vi "Grab SSID Values.vi"(8 "error in (no error)":errorcluster, 11 "standard output":string="SSID 1 : \n    Network type            : Infrastructure\r\n    Authentication          : WPA2-Personal\r\n    Encryption              : CCMP \r\n\r\nSSID 2 : MONU_SIGN_HUB\r\n    Network type            : Infrastructure\r\n    Authentication          : WPA2-Personal\r\n    Encryption              : CCMP \r\n\r\nSSID 3 : UHS-GUEST\r\n    Network type            : Infrastructure\r\n    Authentication          : WPA2-Personal\r\n    Encryption              : CCMP \r\n\r\nSSID 4 : UHS\r\n    Network type            : Infrastructure\r\n    Authentication          : Open\r\n    Encryption              : CCMP \r\n\r\nSSID 5 : MB Hotspot 66929\r\n    Network type            : Infrastructure\r\n    Authentication          : WPA2-Personal\r\n    Encryption              : CCMP \r\n\r\nSSID 6 : MYCAR6741\r\n    Network type            : Infrastructure\r\n    Authentication          : WPA2-Personal\r\n    Encryption              : CCMP \r\n\r\nSSID 7 : Justinƒ?Ts iPhone\r\n    Network type            : Infrastructure\r\n    Authentication          : WPA2-Personal\r\n    Encryption              : CCMP \r\n\r\nSSID 8 : \r\n    Network type            : Infrastructure\r\n    Authentication          : Open\r\n    Encryption              : None \r\n\r\nSSID 9 : InDemand\r\n    Network type            : Infrastructure\r\n    Authentication          : Open\r\n    Encryption              : CCMP \r\n\r\nSSID 10 : RTC-Transit-VLAN\r\n    Network type            : Infrastructure\r\n    Authentication          : WPA2-Personal\r\n    Encryption              : CCMP \r\n\r\n") -> (0 "error out":errorcluster, 1 "SSID Count":i32=9, 3 "SSID Values":T1[](array[typedef])=[{"SSID"="Network", "Pswd?"=FALSE, "Hide?"=FALSE}, {"SSID"="MONU_SIGN_HUB", "Pswd?"=FALSE, "Hide?"=FALSE}, {"SSID"="UHS-GUEST", "Pswd?"=FALSE, "Hide?"=FALSE}, {"SSID"="UHS", "Pswd?"=FALSE, "Hide?"=FALSE}, {"SSID"="MB", "Pswd?"=FALSE, "Hide?"=FALSE}, {"SSID"="MYCAR6741", "Pswd?"=FALSE, "Hide?"=FALSE}, {"SSID"="Justinƒ?Ts", "Pswd?"=FALSE, "Hide?"=FALSE}, {"SSID"="InDemand", "Pswd?"=TRUE, "Hide?"=FALSE}, {"SSID"="RTC-Transit-VLAN", "Pswd?"=FALSE, "Hide?"=FALSE}])   [LabVIEW 2024]
uses:
  Controls/Network.ctl
  <vilib>/Utility/error.llb/Trim Whitespace One-Sided.vi
panel:
  out "length":i32
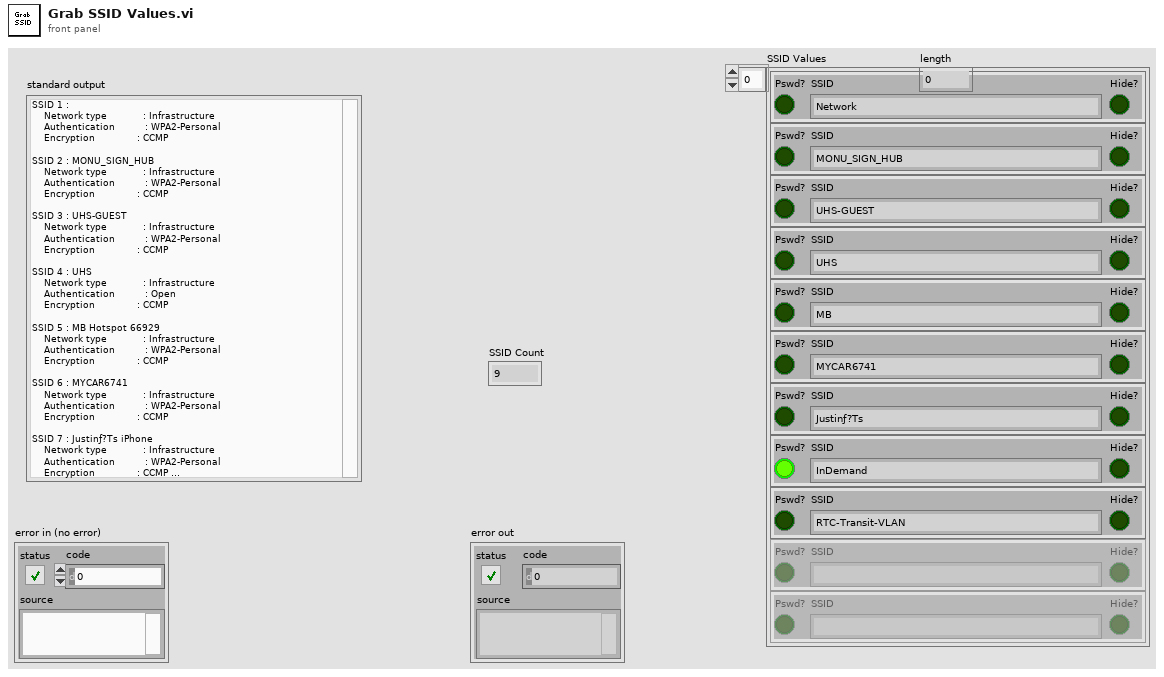
[diagram p1: front panel]
types:
  T1 = typedef "Network.ctl" = cluster{"SSID":string, "Pswd?":bool, "Hide?":bool}
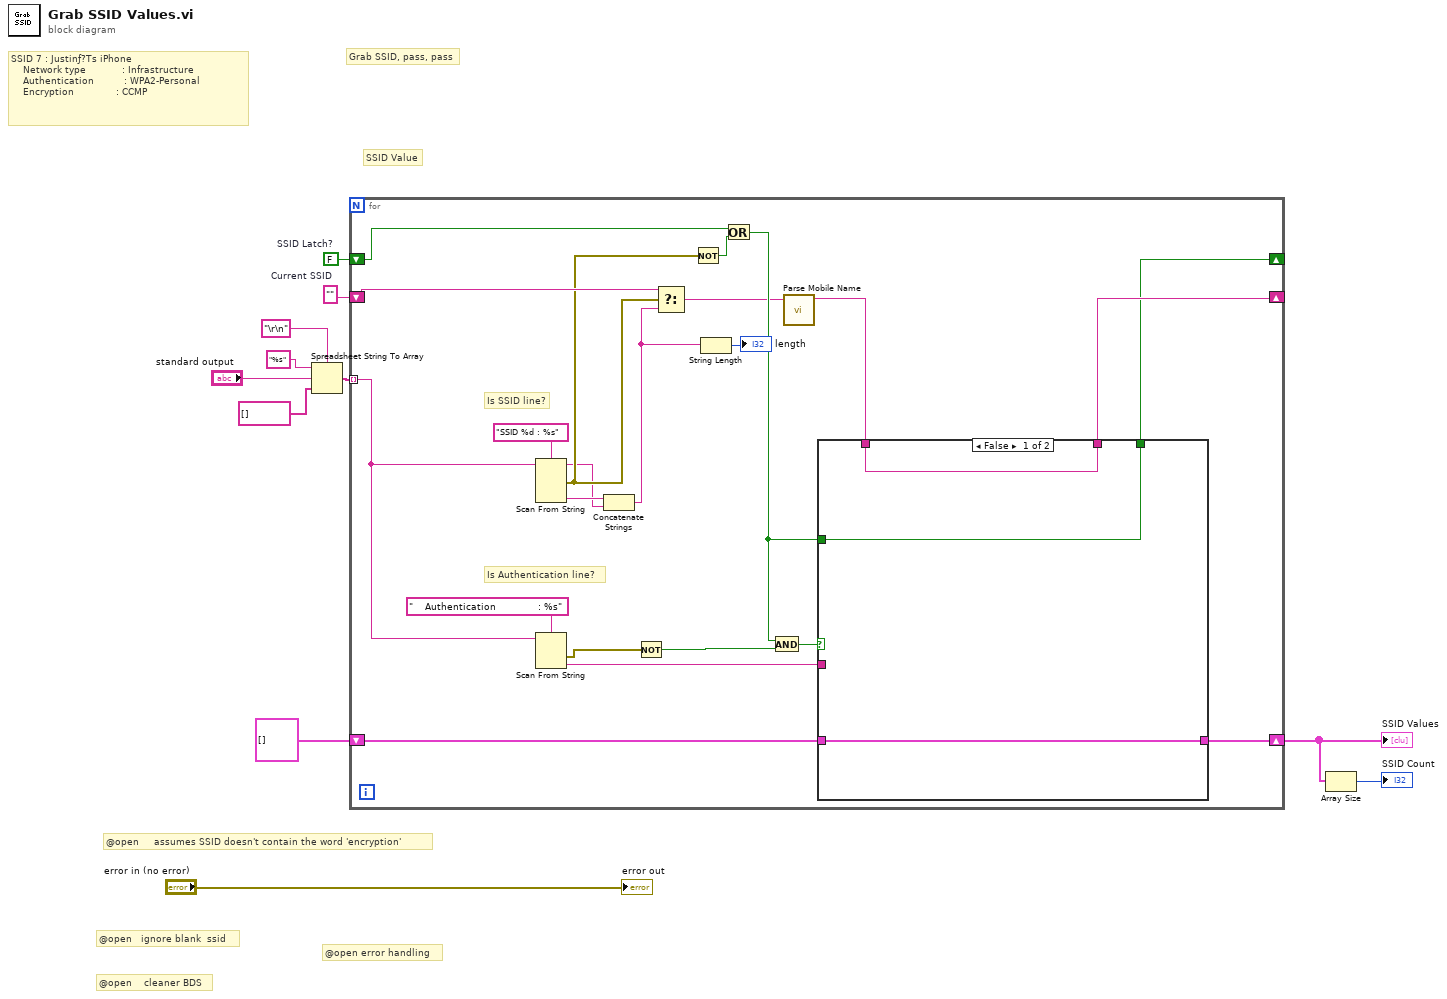
[diagram p0: block diagram]
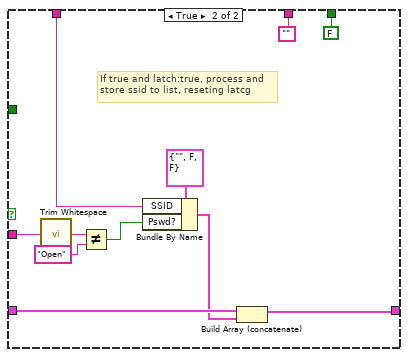
[diagram p2: hidden frame]
diagram:
  w5 = FALSE  # SSID Latch?
  w6 = ""  # Current SSID
  # "@open    cleaner BDS"
  # "@open error handling"
  # "@open   ignore blank  ssid"
  # "@open     assumes SSID doesn't contain the word 'encryption'"
  # "SSID Value"
  # "Grab SSID, pass, pass"
  # "SSID 7 : Justinƒ?Ts iPhone\n    Network type            : Infrastructure\n    Authentication          : WPA2-Personal\n    Encryption              : CCMP"
  n1 = Spreadsheet String To Array(delimiter (Tab)="\r\n", format string="%s", spreadsheet string="standard output", array type (2D Dbl)=string[] []) -> (array=w4:string[])
  n2 = for {
    shift-right: [w27] -> _
    shift-left: w6 -> [w23]
    shift-right: [w26] -> _
    shift-left: w5 -> [w24]
    tunnel: w4 -> [w31] mode=indexing
    shift-right: [w29] -> w2
    shift-left: T1[] [] ("SSID Values 2") -> [w28]
    # "Is Authentication line?"
    # "Is SSID line?"
    n3 = Scan From String(format string="SSID %d : %s", input string=w31) -> (remaining string=w13:string, error out=w17:errorcluster, output 2=w14:string)  [unwired: 5 in, 1 out]
    n4 = Scan From String(format string="    Authentication              : %s", input string=w31) -> (error out=w21:errorcluster, output 1=w19:string)  [unwired: 3 in, 2 out]
    n5 = Concatenate Strings(w14, w13) -> (w12:string)
    n6 = Not(x=w21) -> (.not. x?=w20:bool)
    n7 = Select(t=w23, s=w17, f=w12) -> (s? t:f=w15:string)
    n8 = Not(x=w17) -> (.not. x?=w22:bool)
    n9 = String Length(string=w12) -> (length=→"length":i32)
    n10 = Or(x=w24, y=w22) -> (x .or. y?=w25:bool)
    n11 = And(x=w25, y=w20) -> (x .and. y?=w30:bool)
    n12 = call "Parse Mobile Name.vi"("SSID in"=w15) -> ("SSID out"=w16:string)  [unwired: 8 in, 2 out]
    n13 = case shown="False" w30 {
      tunnel: [w34 w42] -> w29
      tunnel: w28 -> [w34 w43]
      tunnel: w16 -> [w36 w47]
      tunnel: [w36 ""] -> w27
      tunnel: [w35 FALSE] -> w26
      tunnel: w25 -> [w35 _]
      tunnel: w19 -> [_ w41]
      frame False {
      }
      frame True {
        # "If true and latch:true, process and\nstore ssid to list, reseting latcg"
        n14 = call <vilib>:"Trim Whitespace.vi"("string"=w41) -> ("trimmed string"=w39:string)  [unwired: 1 in]
        n15 = Not Equal?(x=w39, y="Open" ("x")) -> (x != y?=w38:bool)
        n16 = Bundle By Name(cluster=T1 {"SSID"="", "Pswd?"=FALSE, "Hide?"=FALSE} ("Network"), "SSID"=w47, "Pswd?"=w38) -> (w37:T1)
        n17 = Build Array (concatenate)(w43, w37) -> (w42:T1[])
      }
    }
  }
  "SSID Values" <- w2
  n18 = Array Size(array=w2) -> (size(s)=→"SSID Count":i32)
  "error out" <- "error in (no error)"
